vi "flattenToString.vi"(8 "error in (no error)":errorcluster, 10 "Record":refnum<class "Record.lvclass">, 11 "Serializer.JSON in":refnum<class "Serializer.JSON.lvclass">) -> (0 "error out":errorcluster, 2 "Flattened String":string, 3 "Serializer.JSON out":refnum<class "Serializer.JSON.lvclass">)   [LabVIEW 2017, in "Serializer.Plug-in.lvlib" / "Serializer.JSON.lvclass"]
uses:
  Serializer.JSON.lvclass
  Record/Record.lvclass
  <vilib>/LabVIEW Open Source Project/OpenSerializer JKI JSON/Serializer.JSON.lvclass
  C:/Program Files (x86)/National Instruments/LabVIEW 2017/vi.lib/LabVIEW Open Source Project/OpenSerializer/Serializer/Serializer.lvclass
  <vilib>/LabVIEW Open Source Project/OpenSerializer/Serializer/Serializer.lvclass
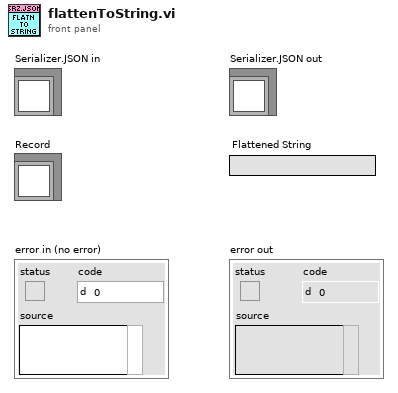
[diagram p1: front panel]
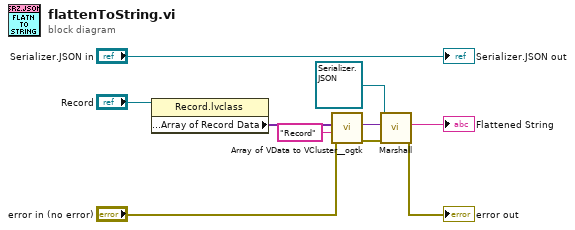
[diagram p0: block diagram]
diagram:
  n1 = property class="Record.lvclass"(reference="Record") -> ("Public API:Properties:Array of Record Data"=w10:variant[])  [unwired: 1 in, 2 out]
  n2 = call <userlib>:"Array of VData to VCluster__ogtk.vi"("error in (no error)"="error in (no error)", "Cluster Name"="Record", "Array"=w10) -> ("error out"=w1:errorcluster, "VCluster"=w8:variant)  [unwired: 7 in]
  n3 = call <vilib>:"Marshall.vi"("error in (no error)"=w1, "Variant"=w8, "Serializer in"=refnum<class "Serializer.JSON.lvclass"> refnum) -> ("error out"=→"error out":errorcluster, "String"=→"Flattened String":string)  [unwired: 6 in, 1 out]
  "Serializer.JSON out" <- "Serializer.JSON in"
